vi "set_up_graph_control_properties.vi"(9 "Graph Properties":T2, 10 "viewing volume":dbl[](array[numeric]), 11 "3D Picture Control Reference":refnum<vi>) -> ()   [LabVIEW 2017, in "3DPC_SurfacePlot.xctl"]
uses:
  <vilib>/Native 3D Graph/xcontrol/3DPC_SurfacePlot.xctl
  <vilib>/Native 3D Graph/typedefs/prop_graph.ctl
  <vilib>/picture/3D Picture Control/NI_3D Picture Control.lvlib
panel:
  in  "View Direction":T1(ring)
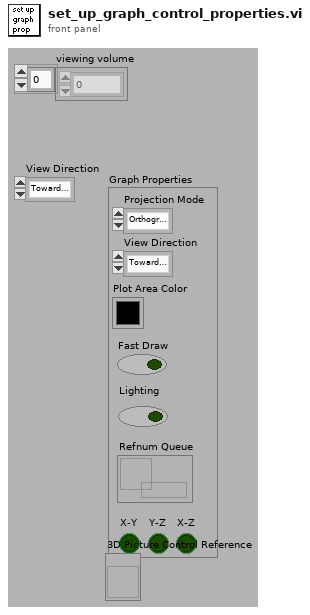
[diagram p1: front panel]
types:
  T1 = enum32{"Towards X-Y Plane", "Towards Y-Z Plane", "Towards X-Z Plane", "User Define"}
  T2 = typedef "3DPC_SurfacePlot.xctl/prop_graph.ctl" = cluster{"Projection Mode":enum16{"Orthographic", "Perspective"}, "View Direction":enum32{"Towards X-Y Plane", "Towards Y-Z Plane", "Towards X-Z Plane", "User Define"}, "Plot Area Color":u32, "Fast Draw":bool, "X-Y":bool, "Y-Z":bool, "X-Z":bool, "Lighting":bool, "Refnum Queue":refnum<queue>}
  T3 = cluster{"Left":sgl, "Left":sgl, "Left":sgl, "Left":sgl, "Left":sgl, "Left":sgl}
  T4 = enum16{"None", "Spherical", "Flying", "Oriented"}
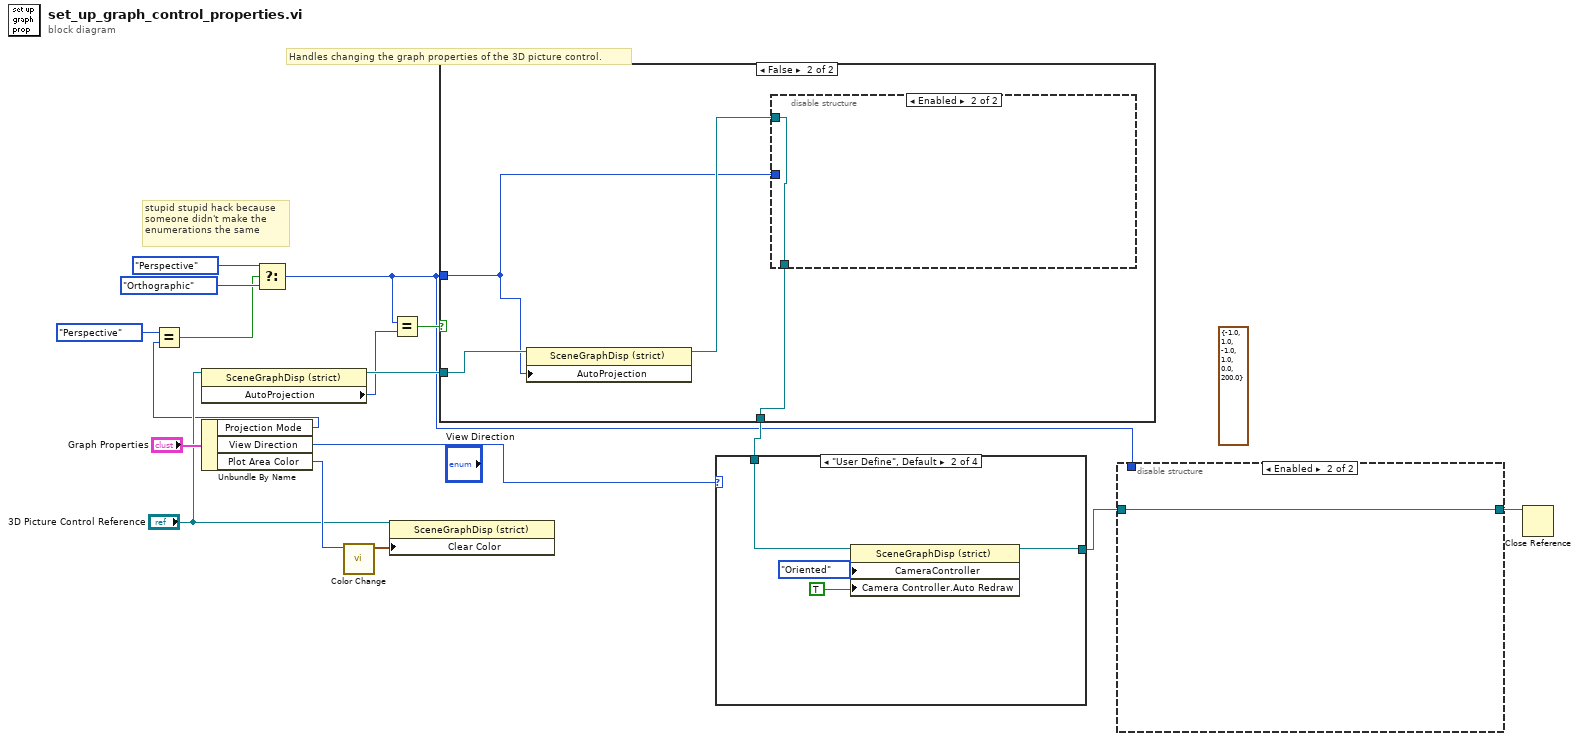
[diagram p0: block diagram]
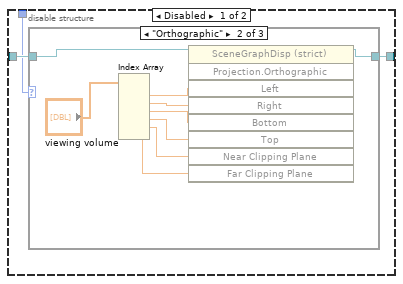
[diagram p2: hidden frame]
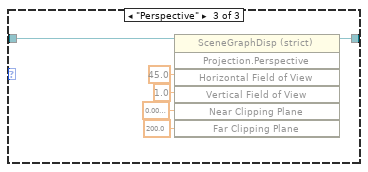
[diagram p4: hidden frame]
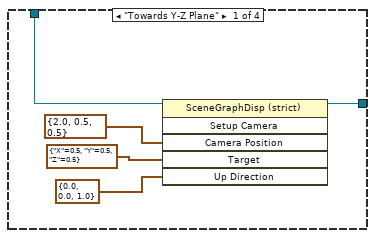
[diagram p5: hidden frame]
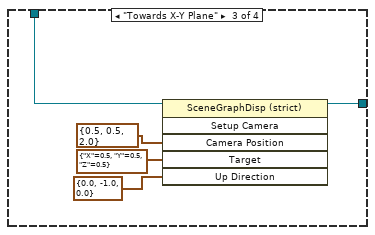
[diagram p6: hidden frame]
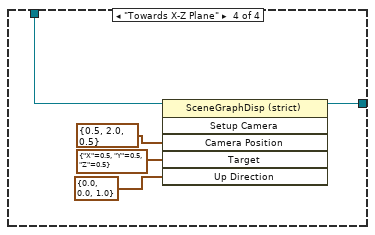
[diagram p7: hidden frame]
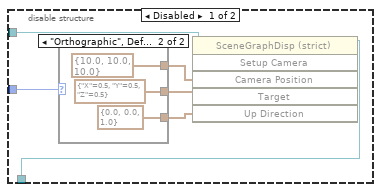
[diagram p9: hidden frame]
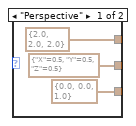
[diagram p10: hidden frame]
diagram:
  (unwired) T3 {"Left"=-1.0, "Left"=1.0, "Left"=-1.0, "Left"=1.0, "Left"=0.0, "Left"=200.0} ("output cluster")
  # "stupid stupid hack because\nsomeone didn't make the \nenumerations the same"
  # "Handles changing the graph properties of the 3D picture control."
  n1 = property class="SceneGraphDisp (strict)"(reference="3D Picture Control Reference") -> (reference out=w11:refnum<vi>, "AutoProjection"=w4:enum16{"None", "Perspective", "Orthographic"})  [unwired: 1 in, 1 out]
  n2 = Unbundle By Name("Graph Properties") -> ("Projection Mode"=w7:enum16{"Orthographic", "Perspective"}, "View Direction"=w16:T1, "Plot Area Color"=w15:u32)
  n3 = Equal?(x=enum16{"Orthographic", "Perspective"}."Perspective", y=w7) -> (x = y?=w5:bool)
  n4 = Select(t=enum16{"None", "Perspective", "Orthographic"}."Perspective" ("Automatic Projection Mode"), s=w5, f=enum16{"None", "Perspective", "Orthographic"}."Orthographic" ("Automatic Projection Mode")) -> (s? t:f=w1:enum16{"None", "Perspective", "Orthographic"})
  n5 = call <vilib>:"Color Change.vi"("Color"=w15) -> ("RGBA"=w14:cluster{"R":sgl, "G":sgl, "B":sgl, "A":sgl})  [unwired: 1 in, 9 out]
  n6 = property on="Property Node" class="SceneGraphDisp (strict)"(reference="3D Picture Control Reference", "Clear Color"=w14) -> ()  [unwired: 1 in, 2 out]
  n7 = Equal?(x=w1, y=w4) -> (x = y?=w13:bool)
  n8 = case shown="False" w13 {
    tunnel: [w18 w19] -> w10
    tunnel: w11 -> [w18 w22]
    tunnel: w1 -> [_ w20]
    frame True {
    }
    frame False {
      n9 = property class="SceneGraphDisp (strict)"(reference=w22, "AutoProjection"=w20) -> (reference out=w21:refnum<vi>)  [unwired: 1 in, 1 out]
      n10 = disable-structure shown="Enabled" {
        disable-tunnel: w21 -> [w28 w35]
        disable-tunnel: w20 -> [w27 _]
        disable-tunnel: [w26 w35] -> w19
        frame Disabled {
          n11 = case shown="\"Orthographic\", Default" w27 {
            tunnel: [cluster{"Z":sgl, "Y":sgl, "X":sgl} {"Z"=0.0, "Y"=0.0, "X"=1.0} cluster{"Z":sgl, "Y":sgl, "X":sgl} {"Z"=0.0, "Y"=0.0, "X"=1.0}] -> w25
            tunnel: [cluster{"X":sgl, "Y":sgl, "Z":sgl} {"X"=0.5, "Y"=0.5, "Z"=0.5} ("Target") cluster{"X":sgl, "Y":sgl, "Z":sgl} {"X"=0.5, "Y"=0.5, "Z"=0.5} ("Target")] -> w24
            tunnel: [cluster{"X":sgl, "Y":sgl, "Z":sgl} {"X"=2.0, "Y"=2.0, "Z"=2.0} ("Up Direction") cluster{"X":sgl, "Y":sgl, "Z":sgl} {"X"=10.0, "Y"=10.0, "Z"=10.0} ("Up Direction")] -> w23
            frame "Perspective" {
            }
            frame "Orthographic", Default {
            }
          }
          n12 = invoke on="Invoke Node" class="SceneGraphDisp (strict)" method="Setup Camera"(reference=w28, "Camera Position"=w23, "Target"=w24, "Up Direction"=w25) -> (reference out=w26:refnum<vi>)  [unwired: 2 in, 5 out]
        }
        frame Enabled {
        }
      }
    }
  }
  n13 = case shown="\"User Define\", Default" w16 {
    tunnel: [w37 w42 w45 w50] -> w3
    tunnel: w10 -> [w36 w43 w46 w51]
    frame "Towards Y-Z Plane" {
      n14 = invoke class="SceneGraphDisp (strict)" method="Setup Camera"(reference=w36, "Camera Position"=cluster{"X":sgl, "Y":sgl, "Z":sgl} {"X"=2.0, "Y"=0.5, "Z"=0.5}, "Target"=cluster{"X":sgl, "Y":sgl, "Z":sgl} {"X"=0.5, "Y"=0.5, "Z"=0.5} ("Camera Position"), "Up Direction"=cluster{"X":sgl, "Y":sgl, "Z":sgl} {"X"=0.0, "Y"=0.0, "Z"=1.0} ("Camera Position")) -> (reference out=w37:refnum<vi>)  [unwired: 2 in, 5 out]
    }
    frame "User Define", Default {
      n15 = property class="SceneGraphDisp (strict)"(reference=w43, "CameraController"=T4."Oriented" ("Camera Controller:Type"), "Camera Controller.Auto Redraw"=TRUE ("Camera Controller:Auto Redraw")) -> (reference out=w42:refnum<vi>)  [unwired: 1 in, 1 out]
    }
    frame "Towards X-Y Plane" {
      n16 = invoke class="SceneGraphDisp (strict)" method="Setup Camera"(reference=w46, "Camera Position"=cluster{"X":sgl, "Y":sgl, "Z":sgl} {"X"=0.5, "Y"=0.5, "Z"=2.0}, "Target"=cluster{"X":sgl, "Y":sgl, "Z":sgl} {"X"=0.5, "Y"=0.5, "Z"=0.5} ("Camera Position"), "Up Direction"=cluster{"X":sgl, "Y":sgl, "Z":sgl} {"X"=0.0, "Y"=-1.0, "Z"=0.0} ("Camera Position")) -> (reference out=w45:refnum<vi>)  [unwired: 2 in, 5 out]
    }
    frame "Towards X-Z Plane" {
      n17 = invoke class="SceneGraphDisp (strict)" method="Setup Camera"(reference=w51, "Camera Position"=cluster{"X":sgl, "Y":sgl, "Z":sgl} {"X"=0.5, "Y"=2.0, "Z"=0.5}, "Target"=cluster{"X":sgl, "Y":sgl, "Z":sgl} {"X"=0.5, "Y"=0.5, "Z"=0.5} ("Camera Position"), "Up Direction"=cluster{"X":sgl, "Y":sgl, "Z":sgl} {"X"=0.0, "Y"=0.0, "Z"=1.0} ("Camera Position")) -> (reference out=w50:refnum<vi>)  [unwired: 2 in, 5 out]
    }
  }
  n18 = disable-structure shown="Enabled" {
    disable-tunnel: w3 -> [w57 w74]
    disable-tunnel: [w56 w74] -> w2
    disable-tunnel: w1 -> [w55 _]
    frame Disabled {
      n19 = case shown="\"Orthographic\"" w55 {
        tunnel: w57 -> [w58 w66 w69]
        tunnel: [w58 w67 w68] -> w56
        frame "None", Default {
        }
        frame "Orthographic" {
          n20 = Index Array(array="viewing volume") -> (element #1=w64:dbl, element #2=w63:dbl, element #3=w62:dbl, element #4=w61:dbl, element #5=w60:dbl, element #6=w59:dbl)  [unwired: 6 in]
          n21 = invoke on="Invoke Node" class="SceneGraphDisp (strict)" method="Projection.Orthographic"(reference=w66, "Left"=w64, "Right"=w63, "Bottom"=w62, "Top"=w61, "Near Clipping Plane"=w60, "Far Clipping Plane"=w59) -> (reference out=w67:refnum<vi>)  [unwired: 2 in, 8 out]
        }
        frame "Perspective" {
          n22 = invoke on="Invoke Node" class="SceneGraphDisp (strict)" method="Projection.Perspective"(reference=w69, "Horizontal Field of View"=sgl 45.0 ("Field of View"), "Vertical Field of View"=sgl 1.0 ("Aspect Ratio"), "Near Clipping Plane"=sgl 0.01, "Far Clipping Plane"=sgl 200.0) -> (reference out=w68:refnum<vi>)  [unwired: 2 in, 6 out]
        }
      }
    }
    frame Enabled {
    }
  }
  n23 = Close Reference(reference=w2) -> ()  [unwired: 1 in, 1 out]
